vi "Launch TLB` Springboard.vi"   [LabVIEW 2022 SP3]
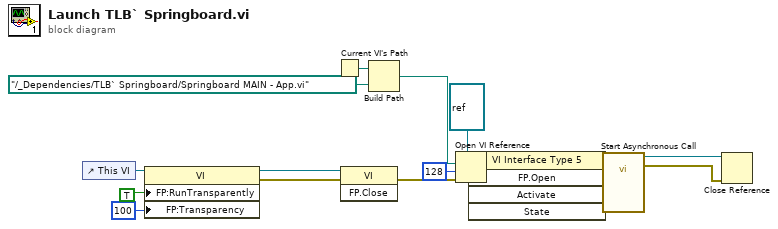
[diagram p0: block diagram]
diagram:
  n1 = control-ref of="This VI"() -> (w12:refnum<vi>)
  n2 = property class="VI"(reference=w12, "FP:RunTransparently"=TRUE ("Front Panel Window:Run VI Transparently"), "FP:Transparency"=u8 100 ("Front Panel Window:Transparency")) -> (reference out=w3:refnum<vi>, error out=w2:errorcluster)  [unwired: 1 in]
  n3 = Current VI's Path() -> (path=w17:path)
  n4 = invoke class="VI" method="FP.Close"(reference=w3, error in=w2) -> (error out=w1:errorcluster)  [unwired: 1 in, 2 out]
  n5 = Build Path(base path=w17, name or relative path=path "../_Dependencies/TLB` Springboard/Springboard MAIN - App.vi" ("vi path")) -> (appended path=w15:path)
  n6 = Open VI Reference(type specifier VI Refnum (for type only)=refnum<vi> refnum, vi path=w15, options=128, error in (no error)=w1) -> (vi reference=w14:refnum<vi>, error out=w13:errorcluster)  [unwired: 2 in]
  n7 = invoke class="VI Interface Type 5" method="FP.Open"(reference=w14, error in=w13) -> (reference out=w9:refnum<vi>, error out=w11:errorcluster)  [unwired: 3 in, 3 out]
  n8 = call-by-ref "Start Asynchronous Call"(reference=w9, error in=w11) -> (reference out=w8:refnum<vi>, error out=w7:errorcluster)  [unwired: 1 in]
  n9 = Close Reference(reference=w8, error in (no error)=w7) -> ()  [unwired: 1 out]
